vi "Identity ID.vi"(11 "DataLoggerIdentity in":refnum<class "DataLoggerIdentity.lvclass">) -> (2 "ID":string)   [LabVIEW 2020, in "Volatus.lvlib" / "DataLoggerIdentity.lvclass"]
uses:
  DataLoggerIdentity.lvclass
  DataLoggerIdentity.lvclass/DataLoggerIdentity.ctl
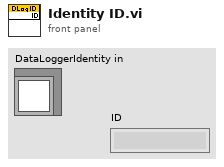
[diagram p1: front panel]
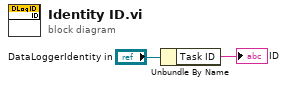
[diagram p0: block diagram]
diagram:
  n1 = Unbundle By Name("DataLoggerIdentity in") -> ("Task ID"=→"ID":string)
